vi "task_2_supp.vi"(11 "Player Info":cluster{"Player1":string, "Score":i32}) -> (3 "Array":cluster{"Player1":string, "Score":i32}[](array[cluster]))   [LabVIEW 2020]
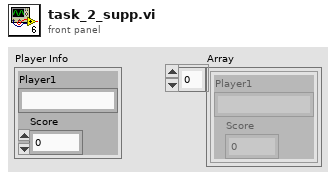
[diagram p1: front panel]
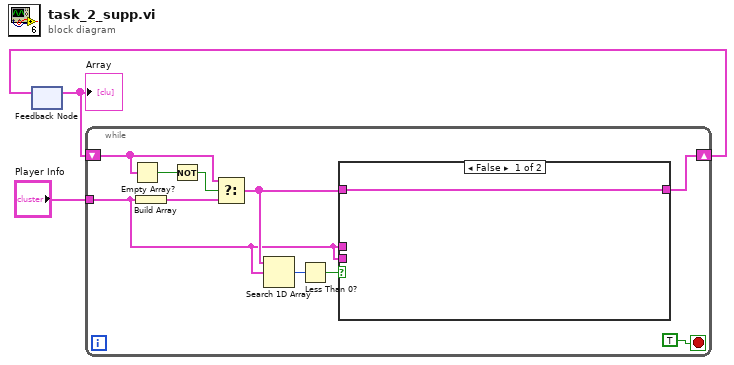
[diagram p0: block diagram]
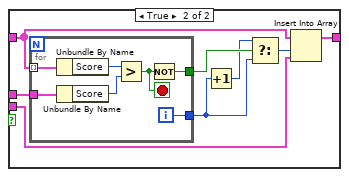
[diagram p2: hidden frame]
diagram:
  n1 = feedback #1() -> (w1:cluster{"Player1":string, "Score":i32}[])  [unwired: 1 in]
  "Array" <- w1
  n2 = while {
    tunnel: "Player Info" -> [w6]
    shift-right: [w7] -> w2
    shift-left: w1 -> [w4]
    stop <- TRUE stop-if-true
    n3 = Empty Array?(array=w4) -> (empty?=w11:bool)
    n4 = Build Array(w6) -> (w13:cluster{"Player1":string, "Score":i32}[])
    n5 = Not(x=w11) -> (.not. x?=w12:bool)
    n6 = Select(t=w4, s=w12, f=w13) -> (s? t:f=w8:cluster{"Player1":string, "Score":i32}[])
    n7 = Search 1D Array(1D array=w8, element=w6) -> (index of element=w10:i32)  [unwired: 1 in]
    n8 = Less Than 0?(x=w10) -> (x < 0?=w9:bool)
    n9 = case shown="False" w9 {
      tunnel: w6 -> [_ w17]
      tunnel: w8 -> [w14 w18]
      tunnel: [w14 w15] -> w7
      tunnel: w6 -> [_ w16]
      frame False {
      }
      frame True {
        n10 = for {
          tunnel: w18 -> [w25] mode=indexing
          tunnel: w16 -> [w27]
          tunnel: [w29] -> w20
          tunnel: [w24] -> w21
          i -> [w29]
          stop <- w23 stop-if-true
          n11 = Unbundle By Name(w25) -> ("Score"=w26:i32)
          n12 = Unbundle By Name(w27) -> ("Score"=w28:i32)
          n13 = Greater?(x=w26, y=w28) -> (0:w23:bool)
          n14 = Not(x=w23) -> (.not. x?=w24:bool)
        }
        n15 = Increment(x=w20) -> (x+1=w19:i32)
        n16 = Select(t=w19, s=w21, f=w20) -> (s? t:f=w22:i32)
        n17 = Insert Into Array(array=w18, index=w22, new element=w17) -> (w15:cluster{"Player1":string, "Score":i32}[])
      }
    }
  }
  n18 = feedback-in #1(w2) -> ()
